vi "Validate Licenece (bidirectional).vi"(8 "error in (no error)":errorcluster, 11 "licence key":string) -> (0 "error out":errorcluster, 2 "features":T1, 3 "licence valid?":bool)   [LabVIEW 2013]
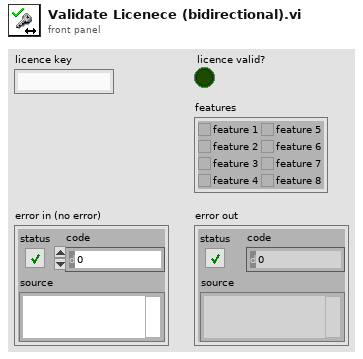
[diagram p1: front panel]
types:
  T1 = cluster{"Feature 1":bool, "Feature 2":bool, "Feature 3":bool, "Feature 4":bool, "Feature 5":bool, "Feature 6":bool, "Feature 7":bool, "Feature 8":bool}
  T2 = cluster{"Boolean array[0]":bool, "Boolean array[1]":bool, "Boolean array[2]":bool, "Boolean array[3]":bool, "Boolean array[4]":bool, "Boolean array[5]":bool, "Boolean array[6]":bool, "Boolean array[7]":bool}
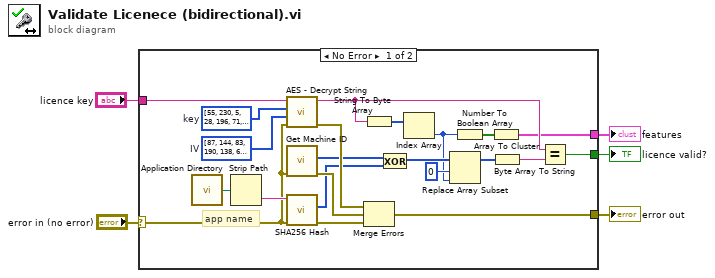
[diagram p0: block diagram]
diagram:
  n1 = case shown="No Error" "error in (no error)" {
    selector: "error in (no error)" -> [w6 w28]
    tunnel: [w10 _] -> w5
    tunnel: [w9 w28] -> w4
    tunnel: "licence key" -> [w8 _]
    tunnel: [w7 _] -> w2
    frame No Error {
      w24 = u8[] [87, 144, 83, 190, 138, 60, 134, 171, 59, 5, 116, 127, 154, 250, 25, 24]  # IV
      w25 = u8[] [55, 230, 5, 28, 196, 71, 246, 204, 4, 31, 53, 16, 0, 203, 136, 242, 182, 15, 199, 174, 127, 6, 27, 184, 229, 147, 86, 4, 208, 54, 91, 185]  # key
      # "app name"
      n2 = call <vilib>:"Application Directory.vi"() -> ("Application Directory"=w23:path)
      n3 = Strip Path(path=w23) -> (name=w22:string)  [unwired: 1 out]
      n4 = call "AES - Decrypt String.vi"("error in (no error)"=w6, "IV"=w24, "key"=w25, "encrypted string"=w8) -> ("error out"=w15:errorcluster, "decrypted string"=w16:string)  [unwired: 6 in]
      n5 = call "Get Machine ID.vi"("error in (no error)"=w6) -> ("error out"=w14:errorcluster, "machine ID bytes"=w11:u8[])  [unwired: 8 in, 1 out]
      n6 = call "SHA256 Hash.vi"("error in (no error)"=w6, "string to hash"=w22) -> ("error out"=w13:errorcluster, "hash bytes"=w12:u8[])  [unwired: 7 in, 1 out]
      n7 = String To Byte Array(string=w16) -> (unsigned byte array=w26:u8[])
      n8 = Merge Errors(w15, w14, w13) -> (w9:errorcluster)
      n9 = Exclusive Or(1:w12, 2:w11) -> (0:w20:u8[])
      n10 = Index Array(array=w26) -> (element=w19:u8)  [unwired: 1 in]
      n11 = Replace Array Subset(array=w20, new element=w19, index=0) -> (w18:u8[])
      n12 = Number To Boolean Array(number=w19) -> (Boolean array=w27:bool[])
      n13 = Array To Cluster(array=w27) -> (cluster=w7:T2)
      n14 = Byte Array To String(unsigned byte array=w18) -> (string=w17:string)
      n15 = Equal?(x=w16, y=w17) -> (x = y?=w10:bool)
    }
    frame Error {
    }
  }
  "error out" <- w4
  "licence valid?" <- w5
  "features" <- w2
